vi "Check Target Resources Channels.vi"(8 "error in":errorcluster, 9 "Target Information in":T1, 10 "tdms file in":refnum<k34>, 11 "Telemetry System Tests in":refnum<class "Telemetry System Tests.lvclass">=refnum) -> (0 "error out":errorcluster, 1 "Target Information out":T1, 2 "tdms file out":refnum<k34>, 3 "Telemetry System Tests out":refnum<class "Telemetry System Tests.lvclass">)   [LabVIEW 2026, in "Telemetry System Tests.lvclass"]
uses:
  Telemetry System Tests.lvclass
  Source/Shared/Constants.vi
  Source/Shared/Telemetry Shared.lvlib
  Source/Engine/Telemetry Engine.lvlib
  <vilib>/NI/VeriStand Custom Device Testing Tools/VeriStandTestUtilities/ChassisInformation.ctl
  <vilib>/NI/VeriStand Custom Device Testing Tools/VeriStandTestUtilities/VeriStandTestUtilities.lvlib
  <vilib>/NI/VeriStand Custom Device Testing Tools/VeriStandTestUtilities/TargetInformation.ctl
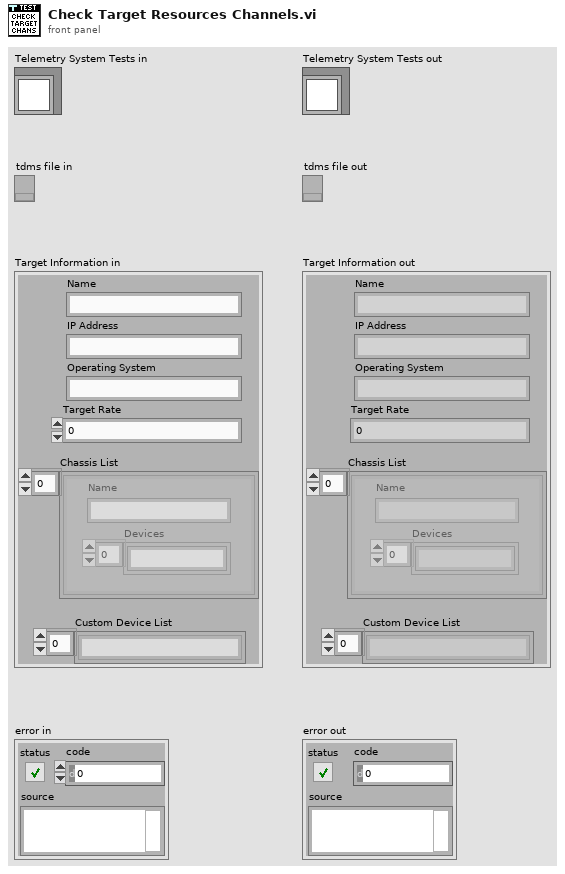
[diagram p1: front panel]
types:
  T1 = typedef "VeriStandTestUtilities.lvlib/TargetInformation.ctl" = cluster{"Name":string, "IP Address":string, "Operating System":string, "Target Rate":dbl, "Chassis List":T2[], "Custom Device List":string[]}
  T2 = typedef "VeriStandTestUtilities.lvlib/ChassisInformation.ctl" = cluster{"Name":string, "Devices":string[]}
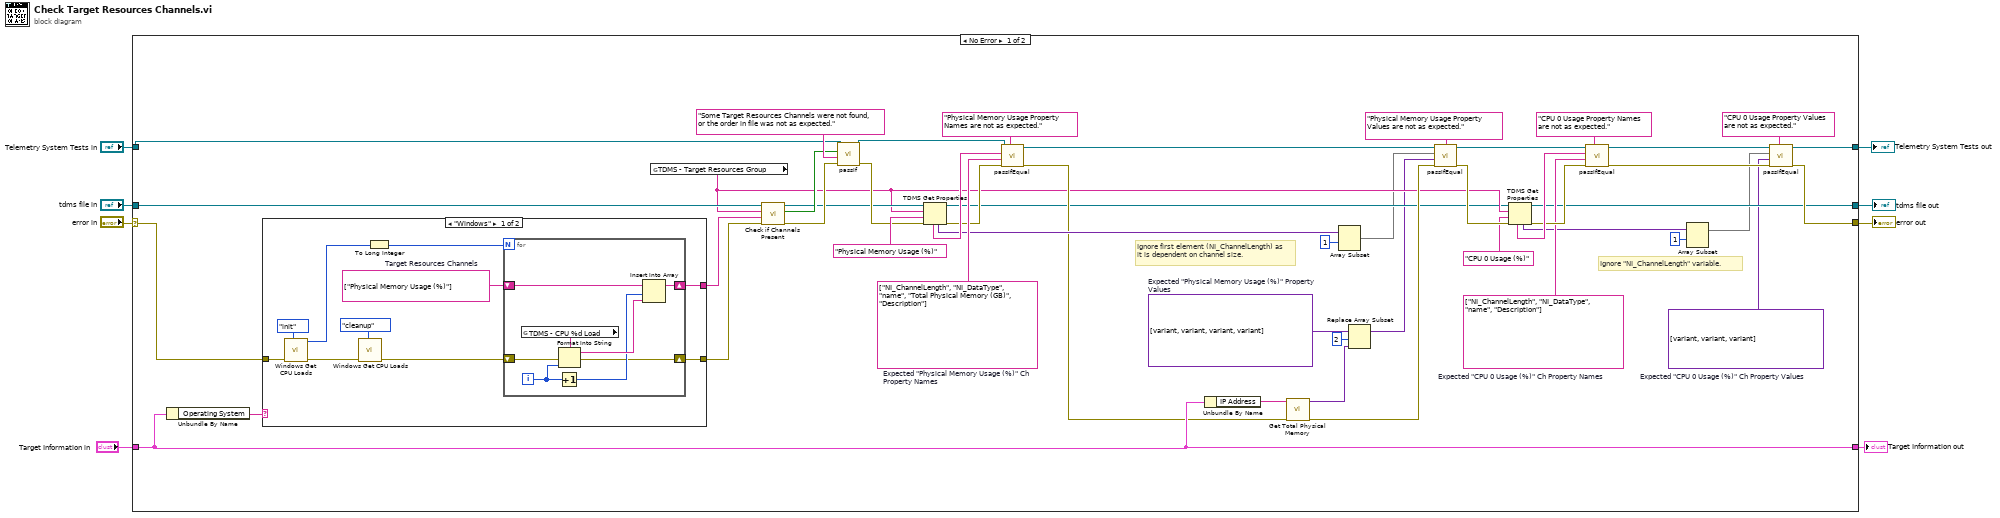
[diagram p0: block diagram]
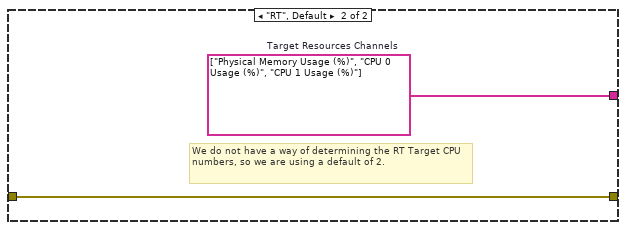
[diagram p2: hidden frame]
diagram:
  n1 = case shown="No Error" "error in" {
    selector: "error in" -> [w40 w81]
    tunnel: [w23 w81] -> w8
    tunnel: [w26 w79] -> w7
    tunnel: [w21 w80] -> w6
    tunnel: "Telemetry System Tests in" -> [w46 w79]
    tunnel: "tdms file in" -> [w44 w80]
    tunnel: "Target Information in" -> [w38 w78]
    tunnel: [w38 w78] -> w1
    frame No Error {
      w11 = variant[] [variant(u16 10), variant(string "Physical Memory Usage (%)"), variant, variant(string "Specifies the amount of used physical memory as a percentage on the system.")]  # Expected "Physical Memory Usage (%)" Property Values
      w17 = variant[] [variant(u16 10), variant(string "CPU 0 Usage (%)"), variant(string "Specifies the total load of the CPU as a percentage on the system.")]  # Expected "CPU 0 Usage (%)" Ch Property Values
      w28 = string[] ["NI_ChannelLength", "NI_DataType", "name", "Description"]  # Expected "CPU 0 Usage (%)" Ch Property Names
      w56 = string[] ["NI_ChannelLength", "NI_DataType", "name", "Total Physical Memory (GB)", "Description"]  # Expected "Physical Memory Usage (%)" Ch Property Names
      # "Ignore first element (NI_ChannelLength) as it is dependent on channel size."
      # "Ignore \"NI_ChannelLength\" variable."
      n2 = Unbundle By Name(w38) -> ("Operating System"=w42:string)
      n3 = case shown="\"Windows\"" w42 {
        tunnel: [w64 w77] -> w41
        tunnel: w40 -> [w66 w76]
        tunnel: [w58 w76] -> w39
        frame "Windows" {
          w65 = string[] ["Physical Memory Usage (%)"]  # Target Resources Channels
          n4 = call "Windows Get CPU Loads.vi"("Action"=enum16{"init", "read", "cleanup"}."init", "error in (no error)"=w66) -> ("error out"=w60:errorcluster, "# of CPUs"=w63:u32)  [unwired: 7 in, 1 out]
          n5 = call "Windows Get CPU Loads.vi"("Action"=enum16{"init", "read", "cleanup"}."cleanup", "error in (no error)"=w60) -> ("error out"=w59:errorcluster)  [unwired: 7 in, 2 out]
          n6 = To Long Integer(number=w63) -> (32bit integer=w62:i32)
          n7 = for {
            N: w62 -> [_]
            shift-right: [w74] -> w64
            shift-left: w65 -> [w75]
            shift-right: [w68] -> w58
            shift-left: w59 -> [w71]
            i -> [w70]
            n8 = global read "Constants.vi" "TDMS - CPU %d Load"() -> (w73:string)
            n9 = Increment(x=w70) -> (x+1=w69:i32)
            n10 = Format Into String(format string=w73, error in=w71, w70) -> (resulting string=w72:string, error out=w68:errorcluster)  [unwired: 1 in]
            n11 = Insert Into Array(array=w75, index=w69, new element=w72) -> (w74:string[])
          }
        }
        frame "RT", Default {
          w77 = string[] ["Physical Memory Usage (%)", "CPU 0 Usage (%)", "CPU 1 Usage (%)"]  # Target Resources Channels
          # "We do not have a way of determining the RT Target CPU numbers, so we are using a default of 2."
        }
      }
      n12 = global read "Constants.vi" "TDMS - Target Resources Group"() -> (w30:string)
      n13 = call "Check if Channels Present.vi"("error in (no error)"=w39, "Channel Names"=w41, "Group name"=w30, "Refnum in"=w44) -> ("error out"=w48:errorcluster, "Passed ?"=w50:bool, "Refnum out"=w45:refnum<k34>)  [unwired: 5 in]
      n14 = call-dynamic "passIf.vi"("error in (no error)"=w48, "message (\"\")"="Some Target Resources Channels were not found, or the order in file was not as expected." ("message (\"\")"), "pass"=w50, "TestCase in"=w46) -> ("error out"=w49:errorcluster, "TestCase out"=w47:refnum<class "Telemetry System Tests.lvclass">)  [unwired: 6 in]
      n15 = TDMS Get Properties(8:w49, 9:"Physical Memory Usage (%)" ("channel name"), 10:w30, 11:w45) -> (0:w54:errorcluster, 3:w22:refnum<k34>, 4:w43:variant[], 6:w57:string[])  [unwired: 2 in, 2 out]
      n16 = call-dynamic "passIfEqual.vi"("custom report message (\"\")"="Physical Memory Usage Property Names are not as expected." ("custom report message (\"\")"), "error in (no error)"=w54, "y"=w56, "x"=w57, "TestCase in"=w47) -> ("error out"=w37:errorcluster, "TestCase out"=w55:refnum<class "Telemetry System Tests.lvclass">)  [unwired: 5 in]
      n17 = Unbundle By Name(w38) -> ("IP Address"=w13:string)
      n18 = call "Get Total Physical Memory.vi"("error in"=w37, "Target IP Address"=w13) -> ("error out"=w36:errorcluster, "Total Physical Memory (GB)"=w9:variant)  [unwired: 8 in]
      n19 = Array Subset(array=w43, index=1) -> (w15:variant[])  [unwired: 1 in]
      n20 = Replace Array Subset(array=w11, new element=w9, index=2) -> (w14:variant[])
      n21 = call-dynamic "passIfEqual.vi"("custom report message (\"\")"="Physical Memory Usage Property Values are not as expected." ("custom report message (\"\")"), "error in (no error)"=w36, "y"=w14, "x"=w15, "TestCase in"=w55) -> ("error out"=w31:errorcluster, "TestCase out"=w32:refnum<class "Telemetry System Tests.lvclass">)  [unwired: 5 in]
      n22 = TDMS Get Properties(8:w31, 9:"CPU 0 Usage (%)" ("channel name"), 10:w30, 11:w22) -> (0:w34:errorcluster, 3:w21:refnum<k34>, 4:w18:variant[], 6:w35:string[])  [unwired: 2 in, 2 out]
      n23 = call-dynamic "passIfEqual.vi"("custom report message (\"\")"="CPU 0 Usage Property Names are not as expected." ("custom report message (\"\")"), "error in (no error)"=w34, "y"=w28, "x"=w35, "TestCase in"=w32) -> ("error out"=w24:errorcluster, "TestCase out"=w27:refnum<class "Telemetry System Tests.lvclass">)  [unwired: 5 in]
      n24 = Array Subset(array=w18, index=1) -> (w20:variant[])  [unwired: 1 in]
      n25 = call-dynamic "passIfEqual.vi"("custom report message (\"\")"="CPU 0 Usage Property Values are not as expected." ("custom report message (\"\")"), "error in (no error)"=w24, "y"=w17, "x"=w20, "TestCase in"=w27) -> ("error out"=w23:errorcluster, "TestCase out"=w26:refnum<class "Telemetry System Tests.lvclass">)  [unwired: 5 in]
    }
    frame Error {
    }
  }
  "error out" <- w8
  "Telemetry System Tests out" <- w7
  "tdms file out" <- w6
  "Target Information out" <- w1
